vi "Disconnect Channel.vi"(8 "error in (no error)":errorcluster, 11 "PXIe 2737 in":refnum<class "PXIe 2737.lvclass">) -> (0 "error out":errorcluster, 3 "PXIe 2737 out":refnum<class "PXIe 2737.lvclass">)   [LabVIEW 2023, in "S-Matrix.lvlib" / "PXIe 2737.lvclass"]
uses:
  PXIe 2737.lvclass
  Abstract/Abstract.lvclass
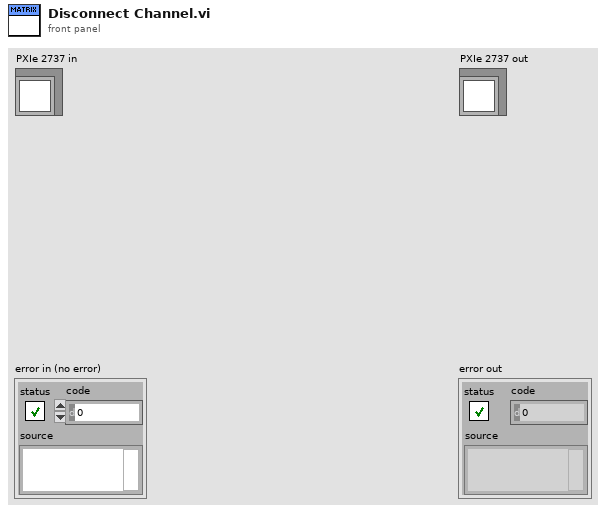
[diagram p1: front panel]
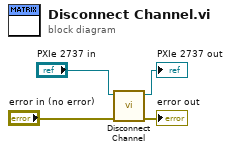
[diagram p0: block diagram]
diagram:
  n1 = call-parent "Disconnect Channel.vi"("error in (no error)"="error in (no error)", "Abstract in"="PXIe 2737 in") -> ("error out"=→"error out":errorcluster, "Abstract out"=→"PXIe 2737 out":refnum<class "PXIe 2737.lvclass">)  [unwired: 8 in]
